vi "Glimpse plugin list plugins.vi"(7 "error in":errorcluster, 10 "stripped path":path) -> (0 "error out":errorcluster, 2 "file names":string[](array[string]), 3 "stripped path out":path)   [LabVIEW 2016]
panel:
  in  "Plug-in paths":path[](array[path])=[path "C:/Users/gelles.USERS/Documents/SVN sandbox/glimpse core/Plug-ins/movie merge/GPI-Movie merge.vi", path "C:/Users/gelles.USERS/Documents/SVN sandbox/glimpse core/Plug-ins/join sequences/GPI-Join Sequences.vi"]
  # "List here plug-ins to be displayed to user as choices.  The file name only\nis used; the path is ignored.  BE SURE TO SET THE VALUES AS DEFAULT \nIF YOU CHANGE THEM.  This list is ONLY used in the executable version;\nsource versions populate the list from all GPI-*.vi files in the same directory\nas the Glimpse-launcher file."
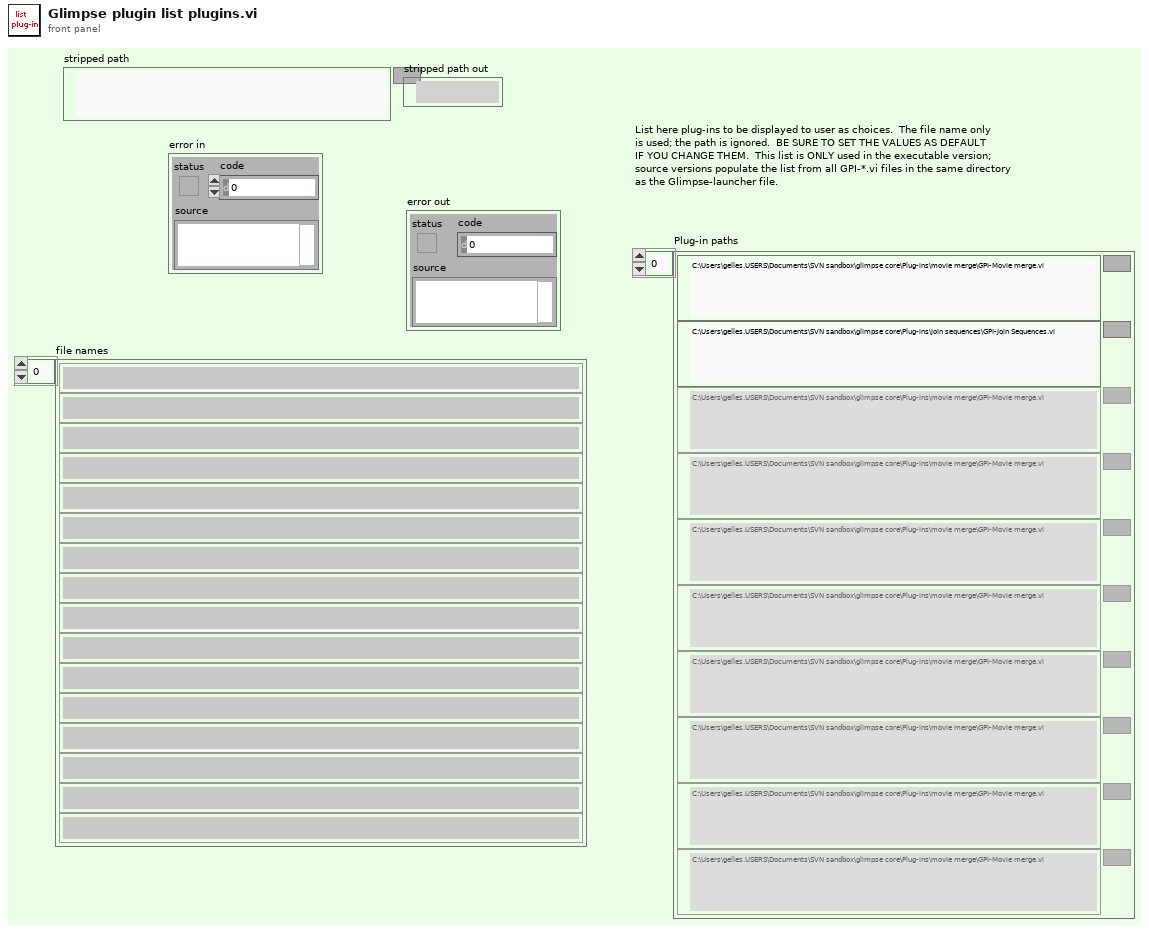
[diagram p1: front panel]
types:
  T1 = enum32{"invalid app kind", "Development System", "Run Time System", "Student Edition", "Embedded LabVIEW", "Evaluation", "Custom"}
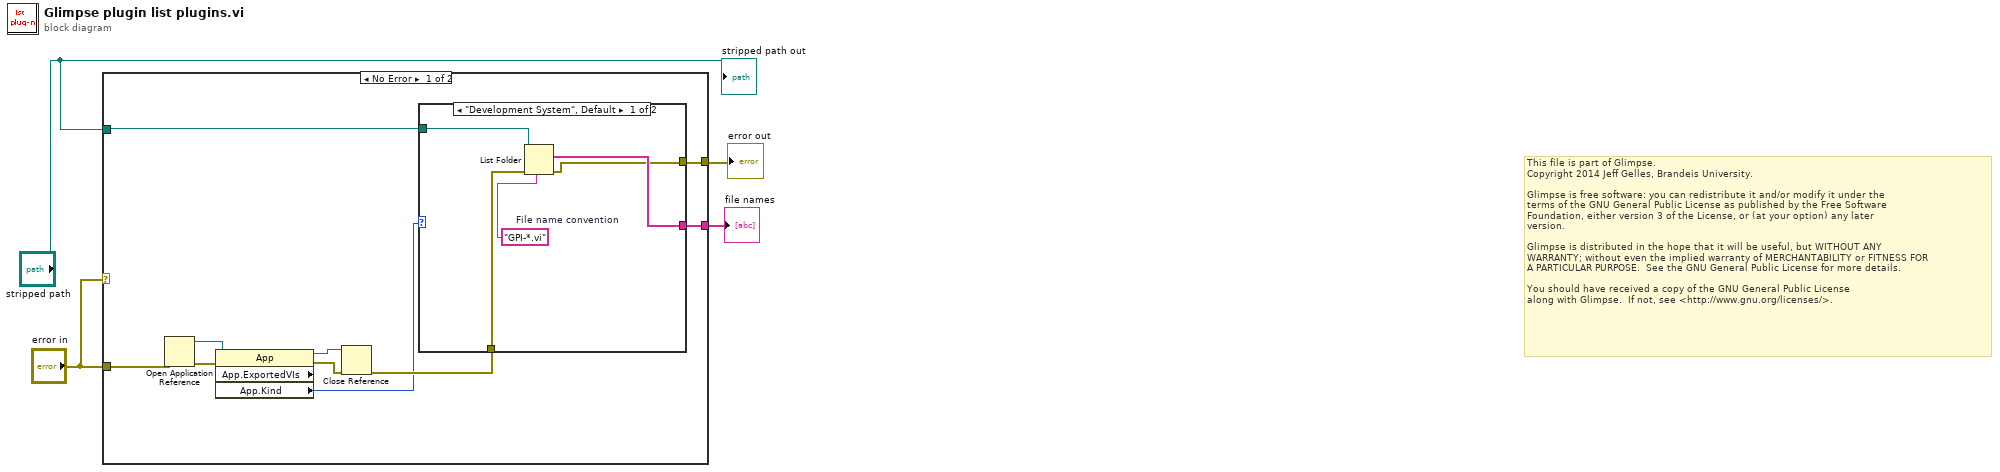
[diagram p0: block diagram]
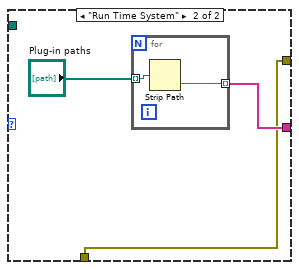
[diagram p2: hidden frame]
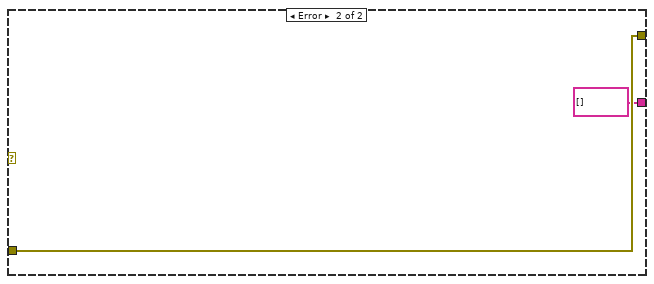
[diagram p3: hidden frame]
diagram:
  # "This file is part of Glimpse. \nCopyright 2014 Jeff Gelles, Brandeis University.    \n\nGlimpse is free software: you can redistribute it and/or modify it under the \nterms of the GNU General Public License as published by the Free Software \nFoundation, either version 3 of the License, or (at your option) any later \nversion.\n\nGlimpse is distributed in the hope that it will be useful, but WITHOUT ANY \nWARRANTY; without even the implied warranty of MERCHANTABILITY or FITNESS FOR \nA PARTICULAR PURPOSE.  See the GNU General Public License for more details.\n\nYou should have received a copy of the GNU General Public License\nalong with Glimpse.  If not, see <http://www.gnu.org/licenses/>."
  n1 = case shown="No Error" "error in" {
    tunnel: "stripped path" -> [w14 _]
    tunnel: [w13 string[] [] ("file names")] -> w3
    tunnel: "error in" -> [w7 w26]
    tunnel: [w12 w26] -> w1
    frame No Error {
      n2 = Open Application Reference(8:w7) -> (0:w10:errorcluster, 3:w11:refnum<vi>)  [unwired: 3 out]
      n3 = property class="App" props=["App.ExportedVIs", "App.Kind"](reference=w11, error in=w10) -> (reference out=w8:refnum<vi>, error out=w9:errorcluster, "App.Kind"=w5:T1)  [unwired: 1 out]
      n4 = Close Reference(reference=w8, error in (no error)=w9) -> (error out=w6:errorcluster)
      n5 = case shown="\"Development System\", Default" w5 {
        tunnel: w14 -> [w19 _]
        tunnel: [w18 w21] -> w13
        tunnel: [w16 w20] -> w12
        tunnel: w6 -> [w15 w20]
        frame "Development System", Default {
          w17 = "GPI-*.vi"  # File name convention
          n6 = List Folder(path=w19, pattern=w17, error in=w15) -> (filenames=w18:string[], error out=w16:errorcluster)  [unwired: 3 out]
        }
        frame "Run Time System" {
          n7 = for {
            tunnel: "Plug-in paths" -> [w24] mode=indexing
            tunnel: [w23] -> w21 mode=indexing
            n8 = Strip Path(path=w24) -> (name=w23:string)  [unwired: 1 out]
          }
        }
      }
    }
    frame Error {
    }
  }
  "file names" <- w3
  "error out" <- w1
  "stripped path out" <- "stripped path"
